vi "UDP Data Link - Configuration Utilities - Get Disable and Symbols.vi"(8 "Mode":enum16{"Tx", "Rx"}(ring), 9 "Channel Type":T1, 10 "Is Channel?":bool, 11 "Is Selected?":bool) -> (1 "Disabled?":bool, 3 "Symbole":i32=1)   [LabVIEW 2015, in "UDP Data Link System Explorer.lvlib"]
doc: "Determines the symbol and enable/disable for a System Definition Channel as displayed within the Channel Selection Dialogs."
uses:
  UDP Data Link System Explorer.lvlib
  <vilib>/NI Veristand/Custom Device API/Custom Device Channel Type.ctl
  <vilib>/NI Veristand/Custom Device API/Custom Device API.lvlib
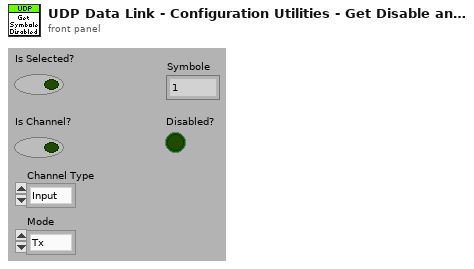
[diagram p1: front panel]
types:
  T1 = typedef "Custom Device API.lvlib/Custom Device Channel Type.ctl" = enum16{"Input", "Output"}
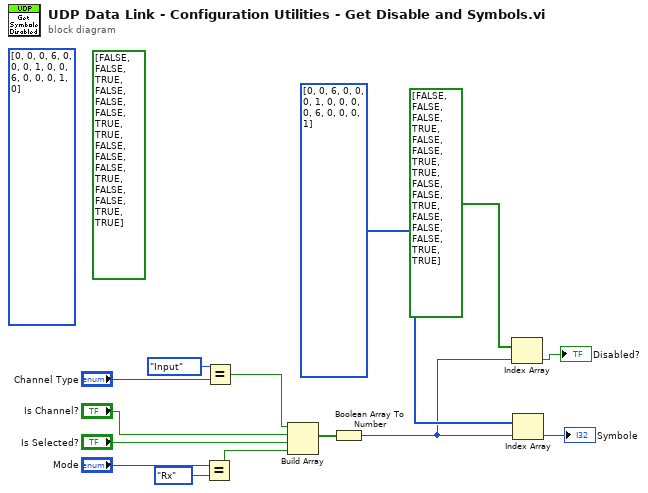
[diagram p0: block diagram]
diagram:
  (unwired) bool[] [FALSE, FALSE, TRUE, FALSE, FALSE, FALSE, TRUE, TRUE, FALSE, FALSE, FALSE, TRUE, FALSE, FALSE, TRUE, TRUE]
  (unwired) i32[] [0, 0, 0, 6, 0, 0, 0, 1, 0, 0, 6, 0, 0, 0, 1, 0]
  n1 = Equal?(x="Mode", y=enum16{"Tx", "Rx"}."Rx") -> (x = y?=w7:bool)
  n2 = Equal?(x=Custom_Device_Channel_Type."Input", y="Channel Type") -> (x = y?=w4:bool)
  n3 = Build Array(w4, "Is Channel?", "Is Selected?", w7) -> (w6:bool[])
  n4 = Boolean Array To Number(Boolean array=w6) -> (number=w1:u32)
  n5 = Index Array(array=bool[] [FALSE, FALSE, FALSE, TRUE, FALSE, FALSE, TRUE, TRUE, FALSE, FALSE, TRUE, FALSE, FALSE, FALSE, TRUE, TRUE], index=w1) -> (element=→"Disabled?":bool)
  n6 = Index Array(array=i32[] [0, 0, 6, 0, 0, 0, 1, 0, 0, 0, 0, 6, 0, 0, 0, 1], index=w1) -> (element=→"Symbole":i32)
